vi "AuMT8852B AFH Active Channel Map.vi"(8 "error in (no error)":errorcluster, 11 "VISA session":refnum<visa-resource-name>) -> (0 "error out":errorcluster, 2 "error code":i32, 3 "VISA session out":refnum<visa-resource-name>, 4 "Active Channel Map":cluster{"Pseudo Local Assessment Map":bool[][]}, 6 "Hex representation of map":string)   [LabVIEW 2017]
doc: "Anritsu MT8852B Bluetooth Tester\n\nProvides a visual and hexadecimal representation of the Active Channel Map used in AFH testing.\n\nOUTPUTS\nActive Channel Map - a visual representation of the Active Channel Map.\nHex representation of map - the hexadecimal string representation of the map."
panel:
  # "0"
  # "10"
  # "20"
  # "30"
  # "40"
  # "50"
  # "60"
  # "70"
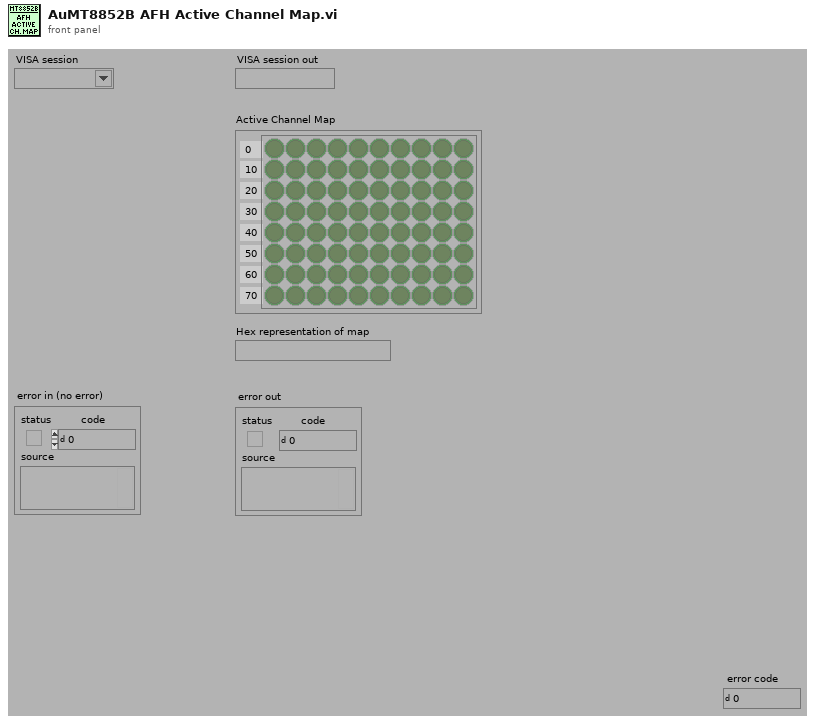
[diagram p1: front panel]
types:
  T1 = enum16{"Simulate", "Range check", "Cache", "Query instrument status"}
  T2 = cluster{"Boolean array[0]":bool, "Boolean array[1]":bool, "Boolean array[2]":bool, "Boolean array[3]":bool, "Boolean array[4]":bool, "Boolean array[5]":bool, "Boolean array[6]":bool, "Boolean array[7]":bool}
  T3 = cluster{"Boolean array[0]":bool, "Boolean array[1]":bool, "Boolean array[2]":bool, "Boolean array[3]":bool, "Boolean array[4]":bool, "Boolean array[5]":bool, "Boolean array[6]":bool}
  T4 = cluster{"Boolean array[0]":bool, "Boolean array[1]":bool, "Boolean array[2]":bool, "Boolean array[3]":bool, "Boolean array[4]":bool, "Boolean array[5]":bool, "Boolean array[6]":bool, "Boolean array[7]":bool, "Boolean array[0]":bool, "Boolean array[1]":bool, "Boolean array[2]":bool, "Boolean array[3]":bool, "Boolean array[4]":bool, "Boolean array[5]":bool, "Boolean array[6]":bool, "Boolean array[7]":bool, "Boolean array[0]":bool, "Boolean array[1]":bool, "Boolean array[2]":bool, "Boolean array[3]":bool, "Boolean array[4]":bool, "Boolean array[5]":bool, "Boolean array[6]":bool, "Boolean array[7]":bool, "Boolean array[0]":bool, "Boolean array[1]":bool, "Boolean array[2]":bool, "Boolean array[3]":bool, "Boolean array[4]":bool, "Boolean array[5]":bool, "Boolean array[6]":bool, "Boolean array[7]":bool, "Boolean array[0]":bool, "Boolean array[1]":bool, "Boolean array[2]":bool, "Boolean array[3]":bool, "Boolean array[4]":bool, "Boolean array[5]":bool, "Boolean array[6]":bool, "Boolean array[7]":bool, "Boolean array[0]":bool, "Boolean array[1]":bool, "Boolean array[2]":bool, "Boolean array[3]":bool, "Boolean array[4]":bool, "Boolean array[5]":bool, "Boolean array[6]":bool, "Boolean array[7]":bool, "Boolean array[0]":bool, "Boolean array[1]":bool, "Boolean array[2]":bool, "Boolean array[3]":bool, "Boolean array[4]":bool, "Boolean array[5]":bool, "Boolean array[6]":bool, "Boolean array[7]":bool, "Boolean array[0]":bool, "Boolean array[1]":bool, "Boolean array[2]":bool, "Boolean array[3]":bool, "Boolean array[4]":bool, "Boolean array[5]":bool, "Boolean array[6]":bool, "Boolean array[7]":bool, "Boolean array[0]":bool, "Boolean array[1]":bool, "Boolean array[2]":bool, "Boolean array[3]":bool, "Boolean array[4]":bool, "Boolean array[5]":bool, "Boolean array[6]":bool, "Boolean array[7]":bool, "Boolean array[0]":bool, "Boolean array[1]":bool, "Boolean array[2]":bool, "Boolean array[3]":bool, "Boolean array[4]":bool, "Boolean array[5]":bool, "Boolean array[6]":bool}
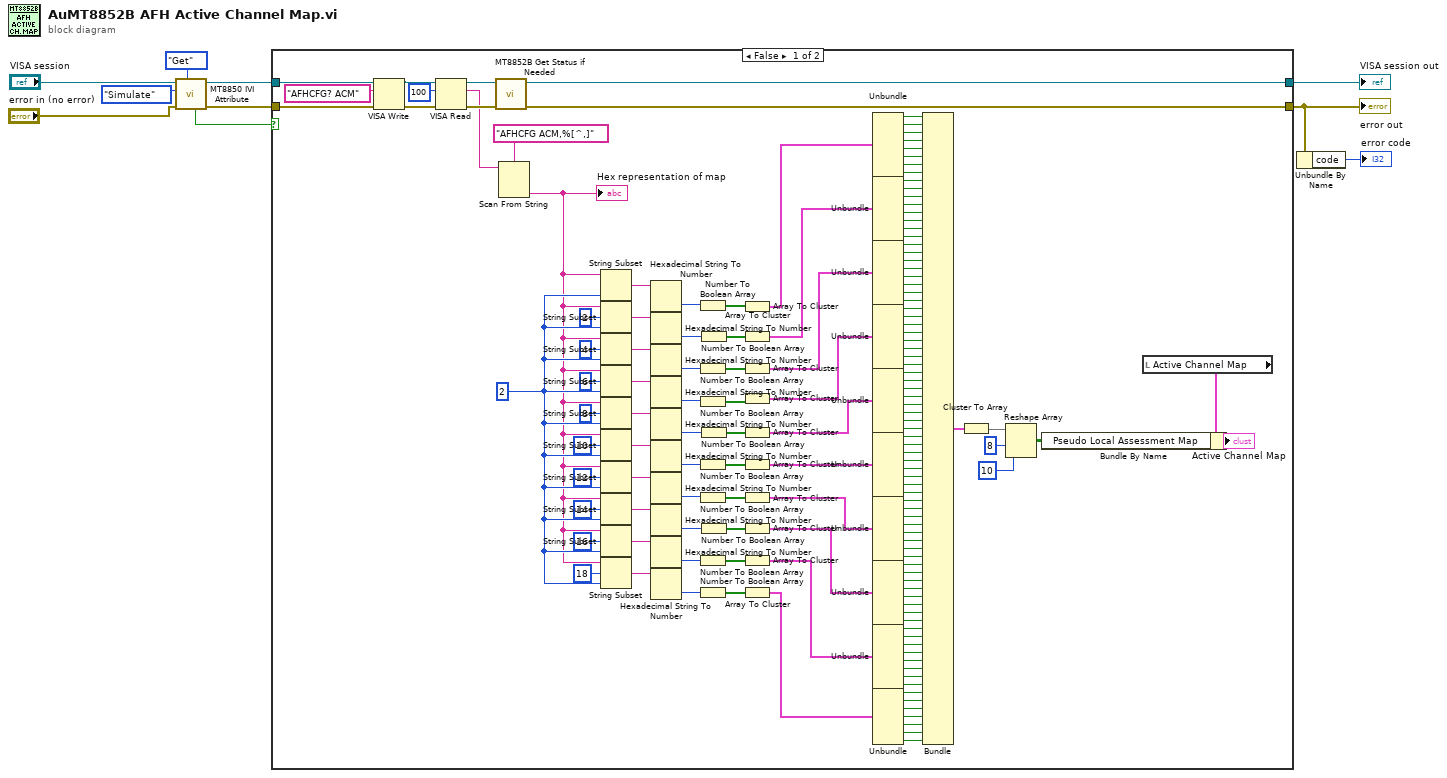
[diagram p0: block diagram]
diagram:
  n1 = call <instrlib>:"MT8850 IVI Attribute.vi"("Set/Get (Set)"=enum16{"Set", "Get"}."Get", "error in (no error)"="error in (no error)", "Flag (Simulate)"=T1."Simulate", "VISA session"="VISA session") -> ("error out"=w9:errorcluster, "VISA session out"=w10:refnum<visa-resource-name>, "Value out"=w6:bool)  [unwired: 5 in]
  n2 = case shown="False" w6 {
    tunnel: [w153 w161] -> w4
    tunnel: [w152 w160] -> w3
    tunnel: w10 -> [w158 w161]
    tunnel: w9 -> [w157 w160]
    frame False {
      w103 = 2 ("length (rest)")
      n3 = VISA Write(VISA resource name=w158, write buffer="AFHCFG? ACM" ("write buffer (\"\")"), error in (no error)=w157) -> (VISA resource name out=w156:refnum<visa-resource-name>, error out=w155:errorcluster)  [unwired: 1 out]
      n4 = VISA Read(VISA resource name=w156, byte count=u32 100 ("byte count (0)"), error in (no error)=w155) -> (VISA resource name out=w150:refnum<visa-resource-name>, read buffer=w149:string, error out=w151:errorcluster)  [unwired: 1 out]
      n5 = call <instrlib>:"MT8852B Get Status if Needed.vi"("error in (no error)"=w151, "VISA session"=w150) -> ("error out"=w152:errorcluster, "VISA session out"=w153:refnum<visa-resource-name>)  [unwired: 8 in]
      n6 = Scan From String(format string="AFHCFG ACM,%[^,]", input string=w149) -> (output 1=w14:string)  [unwired: 3 in, 3 out]
      "Hex representation of map" <- w14
      n7 = String Subset(string=w14, length (rest)=w103) -> (substring=w121:string)  [unwired: 1 in]
      n8 = String Subset(string=w14, offset (0)=2, length (rest)=w103) -> (substring=w120:string)
      n9 = String Subset(string=w14, offset (0)=4, length (rest)=w103) -> (substring=w119:string)
      n10 = String Subset(string=w14, offset (0)=6, length (rest)=w103) -> (substring=w118:string)
      n11 = String Subset(string=w14, offset (0)=8, length (rest)=w103) -> (substring=w117:string)
      n12 = String Subset(string=w14, offset (0)=10, length (rest)=w103) -> (substring=w116:string)
      n13 = String Subset(string=w14, offset (0)=12, length (rest)=w103) -> (substring=w115:string)
      n14 = String Subset(string=w14, offset (0)=14, length (rest)=w103) -> (substring=w114:string)
      n15 = String Subset(string=w14, offset (0)=16, length (rest)=w103) -> (substring=w113:string)
      n16 = String Subset(string=w14, offset (0)=18, length (rest)=w103) -> (substring=w101:string)
      n17 = Hexadecimal String To Number(string=w121) -> (number=w147:u32)  [unwired: 2 in, 1 out]
      n18 = Hexadecimal String To Number(string=w120) -> (number=w146:u32)  [unwired: 2 in, 1 out]
      n19 = Hexadecimal String To Number(string=w119) -> (number=w145:u32)  [unwired: 2 in, 1 out]
      n20 = Hexadecimal String To Number(string=w118) -> (number=w127:u32)  [unwired: 2 in, 1 out]
      n21 = Hexadecimal String To Number(string=w117) -> (number=w126:u32)  [unwired: 2 in, 1 out]
      n22 = Hexadecimal String To Number(string=w116) -> (number=w125:u32)  [unwired: 2 in, 1 out]
      n23 = Hexadecimal String To Number(string=w115) -> (number=w124:u32)  [unwired: 2 in, 1 out]
      n24 = Hexadecimal String To Number(string=w114) -> (number=w123:u32)  [unwired: 2 in, 1 out]
      n25 = Hexadecimal String To Number(string=w113) -> (number=w122:u32)  [unwired: 2 in, 1 out]
      n26 = Hexadecimal String To Number(string=w101) -> (number=w102:u32)  [unwired: 2 in, 1 out]
      n27 = Number To Boolean Array(number=w147) -> (Boolean array=w144:bool[])
      n28 = Number To Boolean Array(number=w145) -> (Boolean array=w143:bool[])
      n29 = Number To Boolean Array(number=w127) -> (Boolean array=w28:bool[])
      n30 = Number To Boolean Array(number=w125) -> (Boolean array=w26:bool[])
      n31 = Number To Boolean Array(number=w124) -> (Boolean array=w25:bool[])
      n32 = Number To Boolean Array(number=w122) -> (Boolean array=w23:bool[])
      n33 = Number To Boolean Array(number=w102) -> (Boolean array=w29:bool[])
      n34 = Number To Boolean Array(number=w146) -> (Boolean array=w142:bool[])
      n35 = Number To Boolean Array(number=w126) -> (Boolean array=w27:bool[])
      n36 = Number To Boolean Array(number=w123) -> (Boolean array=w24:bool[])
      n37 = Array To Cluster(array=w144) -> (cluster=w141:T2)
      n38 = Array To Cluster(array=w142) -> (cluster=w140:T2)
      n39 = Array To Cluster(array=w143) -> (cluster=w139:T2)
      n40 = Array To Cluster(array=w28) -> (cluster=w22:T2)
      n41 = Array To Cluster(array=w27) -> (cluster=w21:T2)
      n42 = Array To Cluster(array=w26) -> (cluster=w20:T2)
      n43 = Array To Cluster(array=w25) -> (cluster=w19:T2)
      n44 = Array To Cluster(array=w24) -> (cluster=w18:T2)
      n45 = Array To Cluster(array=w23) -> (cluster=w17:T2)
      n46 = Array To Cluster(array=w29) -> (cluster=w16:T3)
      n47 = Unbundle(w141) -> ("Boolean array[0]"=w138:bool, "Boolean array[1]"=w137:bool, "Boolean array[2]"=w136:bool, "Boolean array[3]"=w135:bool, "Boolean array[4]"=w134:bool, "Boolean array[5]"=w133:bool, "Boolean array[6]"=w132:bool, "Boolean array[7]"=w131:bool)
      n48 = Unbundle(w140) -> ("Boolean array[0]"=w100:bool, "Boolean array[1]"=w99:bool, "Boolean array[2]"=w98:bool, "Boolean array[3]"=w97:bool, "Boolean array[4]"=w96:bool, "Boolean array[5]"=w95:bool, "Boolean array[6]"=w94:bool, "Boolean array[7]"=w93:bool)
      n49 = Unbundle(w139) -> ("Boolean array[0]"=w92:bool, "Boolean array[1]"=w91:bool, "Boolean array[2]"=w90:bool, "Boolean array[3]"=w89:bool, "Boolean array[4]"=w88:bool, "Boolean array[5]"=w87:bool, "Boolean array[6]"=w86:bool, "Boolean array[7]"=w85:bool)
      n50 = Unbundle(w22) -> ("Boolean array[0]"=w84:bool, "Boolean array[1]"=w83:bool, "Boolean array[2]"=w82:bool, "Boolean array[3]"=w81:bool, "Boolean array[4]"=w80:bool, "Boolean array[5]"=w79:bool, "Boolean array[6]"=w77:bool, "Boolean array[7]"=w78:bool)
      n51 = Unbundle(w21) -> ("Boolean array[0]"=w76:bool, "Boolean array[1]"=w75:bool, "Boolean array[2]"=w74:bool, "Boolean array[3]"=w73:bool, "Boolean array[4]"=w72:bool, "Boolean array[5]"=w71:bool, "Boolean array[6]"=w70:bool, "Boolean array[7]"=w69:bool)
      n52 = Unbundle(w20) -> ("Boolean array[0]"=w68:bool, "Boolean array[1]"=w67:bool, "Boolean array[2]"=w66:bool, "Boolean array[3]"=w65:bool, "Boolean array[4]"=w64:bool, "Boolean array[5]"=w63:bool, "Boolean array[6]"=w62:bool, "Boolean array[7]"=w61:bool)
      n53 = Unbundle(w19) -> ("Boolean array[0]"=w60:bool, "Boolean array[1]"=w59:bool, "Boolean array[2]"=w58:bool, "Boolean array[3]"=w57:bool, "Boolean array[4]"=w56:bool, "Boolean array[5]"=w55:bool, "Boolean array[6]"=w54:bool, "Boolean array[7]"=w53:bool)
      n54 = Unbundle(w18) -> ("Boolean array[0]"=w52:bool, "Boolean array[1]"=w51:bool, "Boolean array[2]"=w50:bool, "Boolean array[3]"=w49:bool, "Boolean array[4]"=w48:bool, "Boolean array[5]"=w47:bool, "Boolean array[6]"=w46:bool, "Boolean array[7]"=w45:bool)
      n55 = Unbundle(w17) -> ("Boolean array[0]"=w44:bool, "Boolean array[1]"=w43:bool, "Boolean array[2]"=w42:bool, "Boolean array[3]"=w41:bool, "Boolean array[4]"=w40:bool, "Boolean array[5]"=w39:bool, "Boolean array[6]"=w38:bool, "Boolean array[7]"=w37:bool)
      n56 = Unbundle(w16) -> ("Boolean array[0]"=w36:bool, "Boolean array[1]"=w35:bool, "Boolean array[2]"=w34:bool, "Boolean array[3]"=w33:bool, "Boolean array[4]"=w32:bool, "Boolean array[5]"=w31:bool, "Boolean array[6]"=w30:bool)
      n57 = Bundle("Boolean array[0]"=w138, "Boolean array[1]"=w137, "Boolean array[2]"=w136, "Boolean array[3]"=w135, "Boolean array[4]"=w134, "Boolean array[5]"=w133, "Boolean array[6]"=w132, "Boolean array[7]"=w131, "Boolean array[0]"=w100, "Boolean array[1]"=w99, "Boolean array[2]"=w98, "Boolean array[3]"=w97, "Boolean array[4]"=w96, "Boolean array[5]"=w95, "Boolean array[6]"=w94, "Boolean array[7]"=w93, "Boolean array[0]"=w92, "Boolean array[1]"=w91, "Boolean array[2]"=w90, "Boolean array[3]"=w89, "Boolean array[4]"=w88, "Boolean array[5]"=w87, "Boolean array[6]"=w86, "Boolean array[7]"=w85, "Boolean array[0]"=w84, "Boolean array[1]"=w83, "Boolean array[2]"=w82, "Boolean array[3]"=w81, "Boolean array[4]"=w80, "Boolean array[5]"=w79, "Boolean array[6]"=w77, "Boolean array[7]"=w78, "Boolean array[0]"=w76, "Boolean array[1]"=w75, "Boolean array[2]"=w74, "Boolean array[3]"=w73, "Boolean array[4]"=w72, "Boolean array[5]"=w71, "Boolean array[6]"=w70, "Boolean array[7]"=w69, "Boolean array[0]"=w68, "Boolean array[1]"=w67, "Boolean array[2]"=w66, "Boolean array[3]"=w65, "Boolean array[4]"=w64, "Boolean array[5]"=w63, "Boolean array[6]"=w62, "Boolean array[7]"=w61, "Boolean array[0]"=w60, "Boolean array[1]"=w59, "Boolean array[2]"=w58, "Boolean array[3]"=w57, "Boolean array[4]"=w56, "Boolean array[5]"=w55, "Boolean array[6]"=w54, "Boolean array[7]"=w53, "Boolean array[0]"=w52, "Boolean array[1]"=w51, "Boolean array[2]"=w50, "Boolean array[3]"=w49, "Boolean array[4]"=w48, "Boolean array[5]"=w47, "Boolean array[6]"=w46, "Boolean array[7]"=w45, "Boolean array[0]"=w44, "Boolean array[1]"=w43, "Boolean array[2]"=w42, "Boolean array[3]"=w41, "Boolean array[4]"=w40, "Boolean array[5]"=w39, "Boolean array[6]"=w38, "Boolean array[7]"=w37, "Boolean array[0]"=w36, "Boolean array[1]"=w35, "Boolean array[2]"=w34, "Boolean array[3]"=w33, "Boolean array[4]"=w32, "Boolean array[5]"=w31, "Boolean array[6]"=w30) -> (w15:T4)  [unwired: 1 in]
      n58 = Cluster To Array(cluster=w15) -> (array=w130:bool[])
      n59 = Reshape Array(w130, 8 ("dimension size"), 10 ("dimension size")) -> (w11:bool[][])
      n60 = local read "Active Channel Map"() -> (w12:cluster{"Pseudo Local Assessment Map":bool[][]})
      n61 = Bundle By Name(cluster=w12, "Pseudo Local Assessment Map"=w11) -> (→"Active Channel Map":cluster{"Pseudo Local Assessment Map":bool[][]})
    }
    frame True {
    }
  }
  "error out" <- w3
  "VISA session out" <- w4
  n62 = Unbundle By Name(w3) -> ("code"=→"error code":i32)
